vi "Clear Sync Pump.vi"(8 "error in (no error)":errorcluster, 11 "Item Ref in":T1 format="%.0x") -> (0 "error out":errorcluster, 3 "Section Ref out":T1 format="%.0x")   [LabVIEW 2015, in "DCM System Explorer.lvlib"]
uses:
  DCM System Explorer.lvlib
  <vilib>/NI Veristand/Custom Device API/Custom Device Item Ref.ctl
  Shared/DCM Constants and GUIDs.vi
  <vilib>/NI Veristand/Custom Device Tools/Custom Device Utility Library/NI VeriStand - Search for Item by Name.vi
  <vilib>/NI Veristand/Custom Device Tools/Custom Device Utility Library/Custom Device Utility Library.lvlib
  <vilib>/NI VeriStand/Custom Device API/Custom Device API.lvlib
  DCM Shared.lvlib
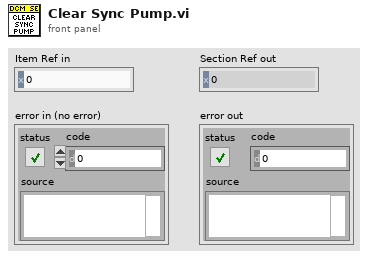
[diagram p1: front panel]
types:
  T1 = typedef "Custom Device API.lvlib/Custom Device Item Ref.ctl" = u64
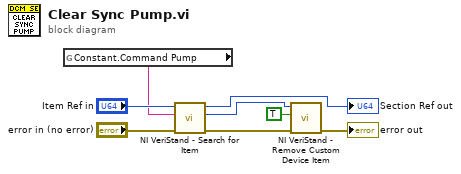
[diagram p0: block diagram]
diagram:
  n1 = global read "DCM Constants and GUIDs.vi" "Constant.Command Pump"() -> (w1:string)
  n2 = call-poly <vilib>:"NI VeriStand - Search for Item.vi"("error in"="error in (no error)", "Item Name"=w1, "Section Ref in"="Item Ref in") -> ("error out"=w5:errorcluster, "Item Ref"=w2:T1, "Section Ref out"=→"Section Ref out":T1)  [unwired: 5 in, 1 out]
  n3 = call <vilib>:"NI VeriStand - Remove Custom Device Item.vi"("error in (no error)"=w5, "Force Delete (F)"=TRUE, "Item Ref in"=w2) -> ("error out"=→"error out":errorcluster)  [unwired: 7 in, 1 out]
